vi "load_SS_compensator_data.vi"(8 "error in (no error)":errorcluster, 11 "Path":path=path "C:/Users/arnold/Documents/afm-cs/labview/UnitTests/fpga_harnesses/SS_Compensators/model.csv") -> (0 "error out":errorcluster, 1 "PHI_square":dbl[][](array[numeric]), 2 "PHI_col":dbl[](array[numeric]), 3 "Ns_1":i32)   [LabVIEW 2017]
uses:
  <vilib>/Utility/error.llb/DialogType.ctl
  <vilib>/Utility/file.llb/Read Delimited Spreadsheet (DBL).vi
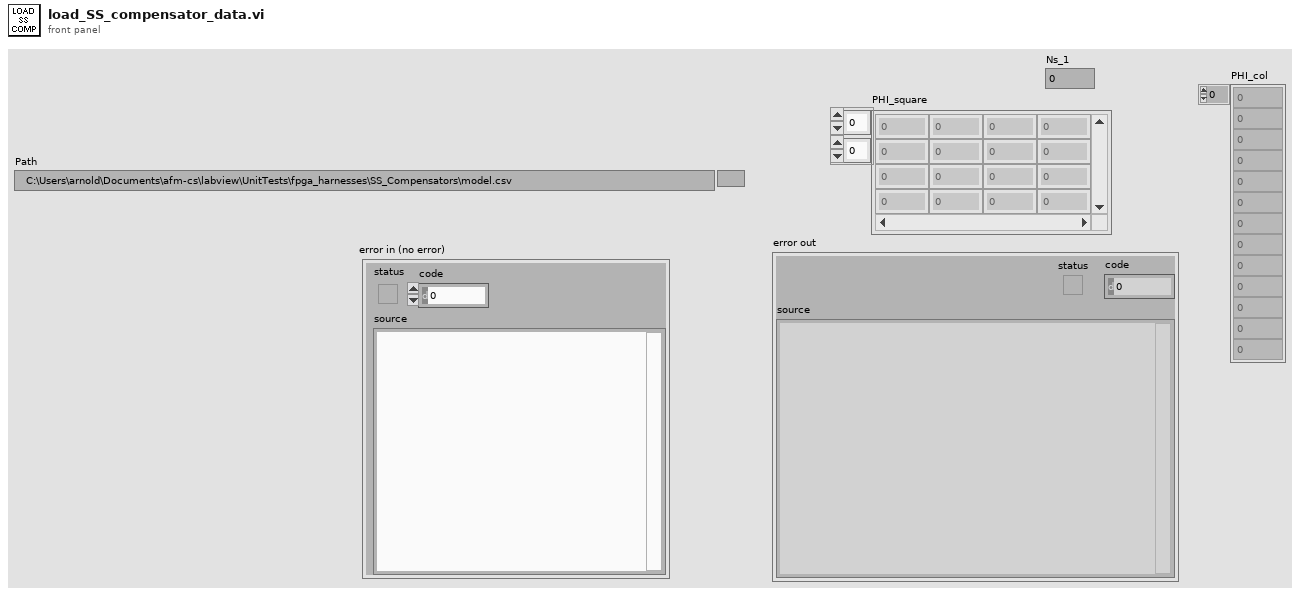
[diagram p1: front panel]
types:
  T1 = typedef "DialogType.ctl" = u16
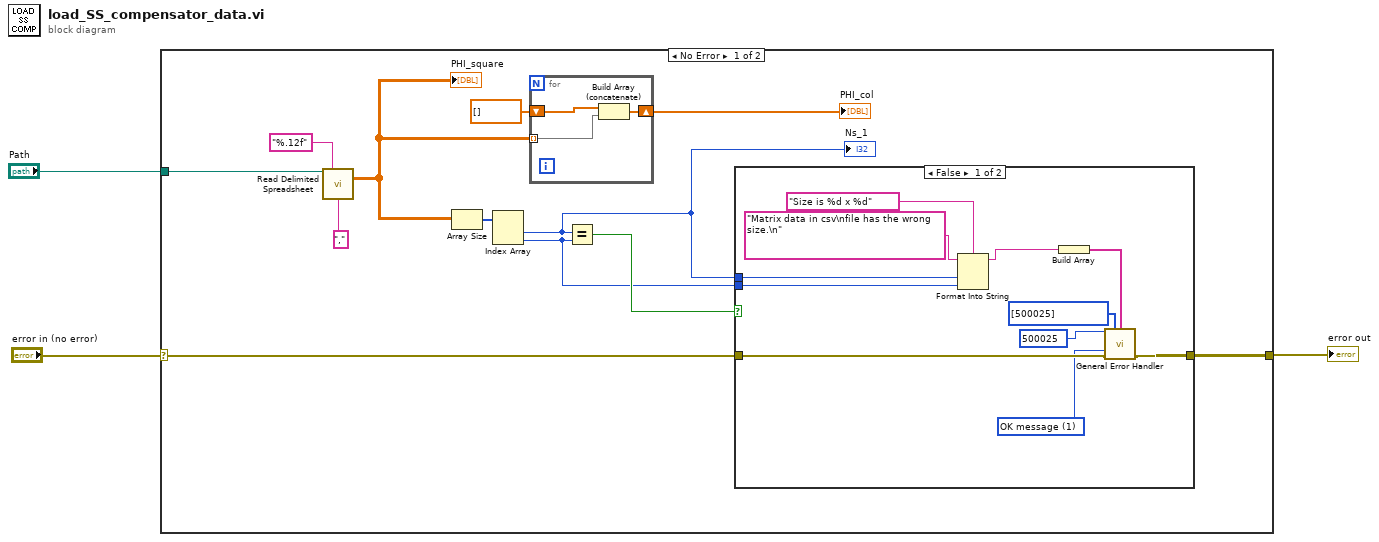
[diagram p0: block diagram]
diagram:
  n1 = case shown="No Error" "error in (no error)" {
    selector: "error in (no error)" -> [w6 w31]
    tunnel: [w9 w31] -> w3
    tunnel: "Path" -> [w8 _]
    frame No Error {
      n2 = call-poly <vilib>:"Read Delimited Spreadsheet.vi"("file path (dialog if empty)"=w8, "format (%.3f)"="%.12f", "delimiter (\\t)"="," ("delimiter (\\t)")) -> ("all rows"=w11:dbl[][])  [unwired: 7 in, 5 out]
      "PHI_square" <- w11
      n3 = Array Size(array=w11) -> (size(s)=w10:i32[])
      n4 = Index Array(array=w10) -> (element #1=w5:i32, element #2=w4:i32)  [unwired: 2 in]
      "Ns_1" <- w5
      n5 = for {
        shift-right: [w30] -> w13
        shift-left: dbl[] [] -> [w29]
        tunnel: w11 -> [w28] mode=indexing
        n6 = Build Array (concatenate)(w29, w28) -> (w30:dbl[])
      }
      "PHI_col" <- w13
      n7 = Equal?(x=w5, y=w4) -> (x = y?=w7:bool)
      n8 = case shown="False" w7 {
        tunnel: [w25 w27] -> w9
        tunnel: w6 -> [w26 w27]
        tunnel: w4 -> [w18 _]
        tunnel: w5 -> [w19 _]
        frame False {
          w23 = T1 1 items=["no dialog", "OK message", "continue or stop message", "OK message + warnings", "continue/stop + warnings"] ("type of dialog (OK msg:1)")
          n9 = Format Into String(format string="Size is %d x %d", initial string="Matrix data in csv\nfile has the wrong size.\n", w19, w18) -> (resulting string=w16:string)  [unwired: 1 in, 1 out]
          n10 = Build Array(w16) -> (w24:string[])
          n11 = call <vilib>:"General Error Handler.vi"("[error code] (0)"=500025, "[user-defined codes]"=i32[] [500025], "[user-defined descriptions]"=w24, "type of dialog (OK msg:1)"=w23, "error in (no error)"=w26) -> ("error out"=w25:errorcluster)  [unwired: 6 in, 4 out]
        }
        frame True {
        }
      }
    }
    frame Error {
    }
  }
  "error out" <- w3
